vi "Load Subpanel VI.vi"(8 "error in":errorcluster, 9 "layout keyword":string, 10 "subpanel VI path":path, 11 "subpanel refnum":refnum<vi>) -> (0 "error out":errorcluster)   [LabVIEW 2012]
uses:
  vi.lib/Front Panel Layout/NI_SE_Front Panel Layout.lvlib
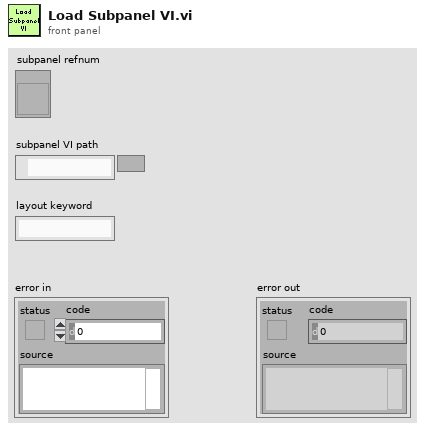
[diagram p1: front panel]
types:
  T1 = typedef "LVBoundsTypeDef.ctl" = cluster{"Width":u32, "Height":u32}
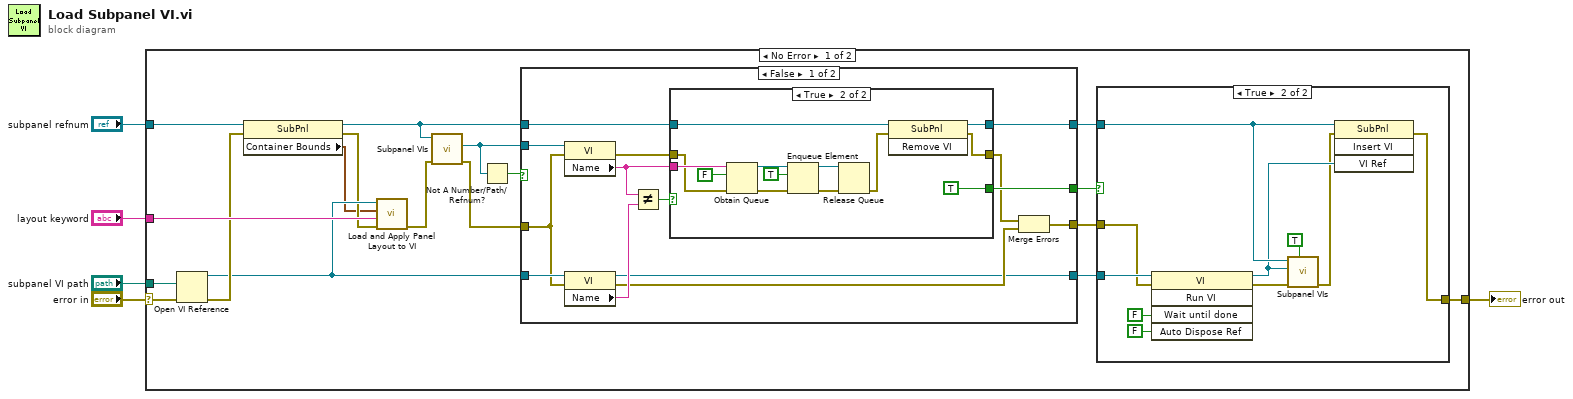
[diagram p0: block diagram]
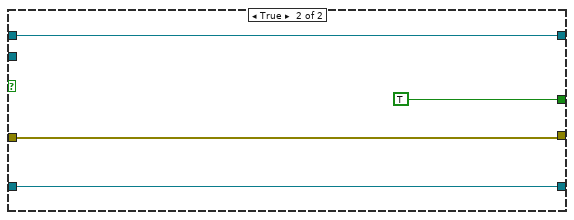
[diagram p4: hidden frame]
diagram:
  n1 = case shown="No Error" "error in" {
    selector: "error in" -> [w23 w68]
    tunnel: [w13 w68] -> w4
    tunnel: "subpanel VI path" -> [w22 _]
    tunnel: "layout keyword" -> [w21 _]
    tunnel: "subpanel refnum" -> [w11 _]
    frame No Error {
      n2 = Open VI Reference(vi path=w22, error in (no error)=w23) -> (vi reference=w18:refnum<vi>, error out=w20:errorcluster)  [unwired: 4 in]
      n3 = property class="SubPnl"(reference=w11, error in=w20) -> (reference out=w10:refnum<vi>, error out=w17:errorcluster, "Container Bounds"=w6:T1)
      n4 = call "Load and Apply Panel Layout to VI.vi"("error in"=w17, "keyword to match (\"\")"=w21, "desired panel size ([-1,-1])"=w6, "VI refnum"=w18) -> ("error out"=w8:errorcluster)  [unwired: 6 in, 1 out]
      n5 = call "Subpanel VIs.vi"("error in"=w8, "subpanel refnum"=w10) -> ("error out"=w7:errorcluster, "subpanel VI out"=w9:refnum<vi>)  [unwired: 8 in]
      n6 = Not A Number/Path/Refnum?(number/path/refnum=w9) -> (NaN/Path/Refnum?=w19:bool)
      n7 = case shown="False" w19 {
        tunnel: w9 -> [w48 _]
        tunnel: w18 -> [w47 w65]
        tunnel: w10 -> [w44 w64]
        tunnel: w7 -> [w40 w67]
        tunnel: [w41 TRUE] -> w12
        tunnel: [w37 w67] -> w15
        tunnel: [w36 w65] -> w16
        tunnel: [w35 w64] -> w14
        frame False {
          n8 = property class="VI"(reference=w48, error in=w40) -> (error out=w42:errorcluster, "Name"=w45:string)  [unwired: 1 out]
          n9 = property class="VI"(reference=w47, error in=w40) -> (reference out=w36:refnum<vi>, error out=w38:errorcluster, "Name"=w46:string)
          n10 = Not Equal?(x=w45, y=w46) -> (x != y?=w43:bool)
          n11 = case shown="True" w43 {
            tunnel: w45 -> [_ w57]
            tunnel: w44 -> [w49 w56]
            tunnel: w42 -> [w50 w55]
            tunnel: [_ TRUE] -> w41
            tunnel: [w50 w52] -> w39
            tunnel: [w49 w51] -> w35
            frame False {
            }
            frame True {
              n12 = Obtain Queue(name (unnamed)=w57, element data type=FALSE, error in (no error)=w55) -> (queue out=w62:refnum<queue>, error out=w61:errorcluster)  [unwired: 2 in, 1 out]
              n13 = Enqueue Element(queue=w62, element=TRUE, error in (no error)=w61) -> (queue out=w59:refnum<queue>, error out=w58:errorcluster)  [unwired: 1 in, 1 out]
              n14 = Release Queue(queue=w59, error in (no error)=w58) -> (error out=w54:errorcluster)  [unwired: 1 in, 2 out]
              n15 = invoke class="SubPnl" method="Remove VI"(reference=w56, error in=w54) -> (reference out=w51:refnum<vi>, error out=w52:errorcluster)  [unwired: 1 in, 1 out]
            }
          }
          n16 = Merge Errors(w39, w38) -> (w37:errorcluster)
        }
        frame True {
        }
      }
      n17 = case shown="True" w12 {
        tunnel: w16 -> [_ w32]
        tunnel: w15 -> [w24 w31]
        tunnel: w14 -> [_ w29]
        tunnel: [w24 w30] -> w13
        frame False {
        }
        frame True {
          n18 = invoke class="VI" method="Run VI"(reference=w32, error in=w31, "Wait until done"=FALSE ("Wait Until Done"), "Auto Dispose Ref"=FALSE ("Auto Dispose Reference")) -> (reference out=w28:refnum<vi>, error out=w26:errorcluster)  [unwired: 1 in, 3 out]
          n19 = call "Subpanel VIs.vi"("write (F)"=TRUE, "error in"=w26, "subpanel VI in"=w28, "subpanel refnum"=w29) -> ("error out"=w25:errorcluster)  [unwired: 6 in, 1 out]
          n20 = invoke class="SubPnl" method="Insert VI"(reference=w29, error in=w25, "VI Ref"=w28) -> (error out=w30:errorcluster)  [unwired: 1 in, 3 out]
        }
      }
    }
    frame Error {
    }
  }
  "error out" <- w4
